vi "PLZ164WA_main.vi"() -> ()   [LabVIEW 2016]
doc: "Demonstrates the usage of major configuration controls. It configures the range, values, input and protection limits."
uses:
  <vilib>/Utility/file.llb/Read Delimited Spreadsheet (DBL).vi
  <instrlib>/Kikusui PLZ 4W Series/Kikusui PLZ 4W Series.lvlib
panel:
  in  "Stop VI":bool
  in  "file path":path=path "C:/Repository/bdc_prototype/logger/new_current_profile.csv"
  in  "Serial Configuration":cluster{"Baud Rate":u32, "Stop Bits":u16}={"Baud Rate"=19200, "Stop Bits"=20} {"Stop Bits" items=["1.0"=10, "2.0"=20]; "Baud Rate" items=["2400"=2400, "4800"=4800, "9600"=9600, "19200"=19200]}
  in  "OPP Trip (Disable)":bool=TRUE
  in  "OCP Trip (Disable)":bool=TRUE
  in  "UVP (Enable)":bool
  in  "Enable Input Short (Disable)":bool
  in  "Enable Input (Enable)":bool=TRUE
  in  "UVP Limit (0)":dbl
  in  "OPP Limit (0)":dbl=5.0
  in  "OCP Limit (0)":dbl=3.0
  in  "VISA resource name":refnum<visa-resource-name>="USB0::0x0B3E::0x1019::YL002399::INSTR"
  # "(c) 2009  National Instruments.  ALL RIGHTS RESERVED."
  # "Input Controls"
  # "Input Protection Controls"
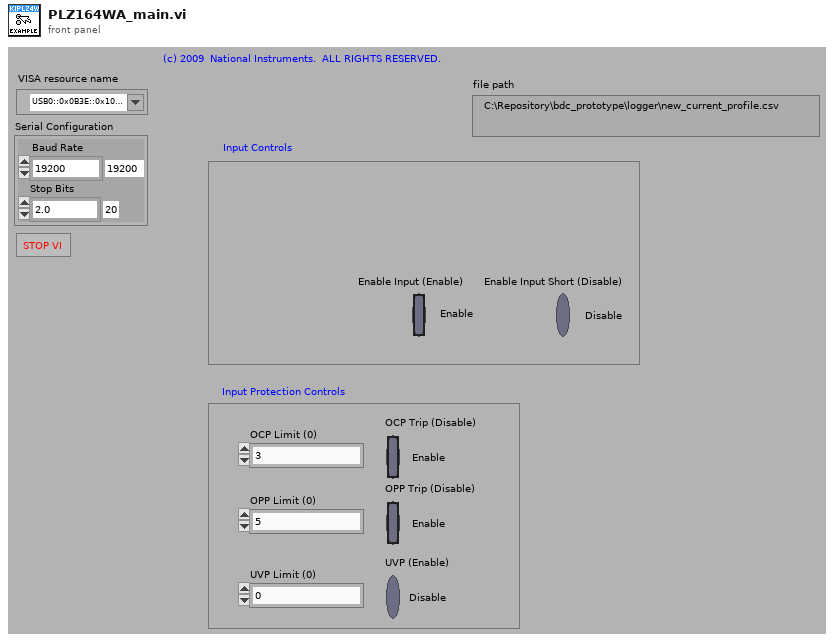
[diagram p1: front panel]
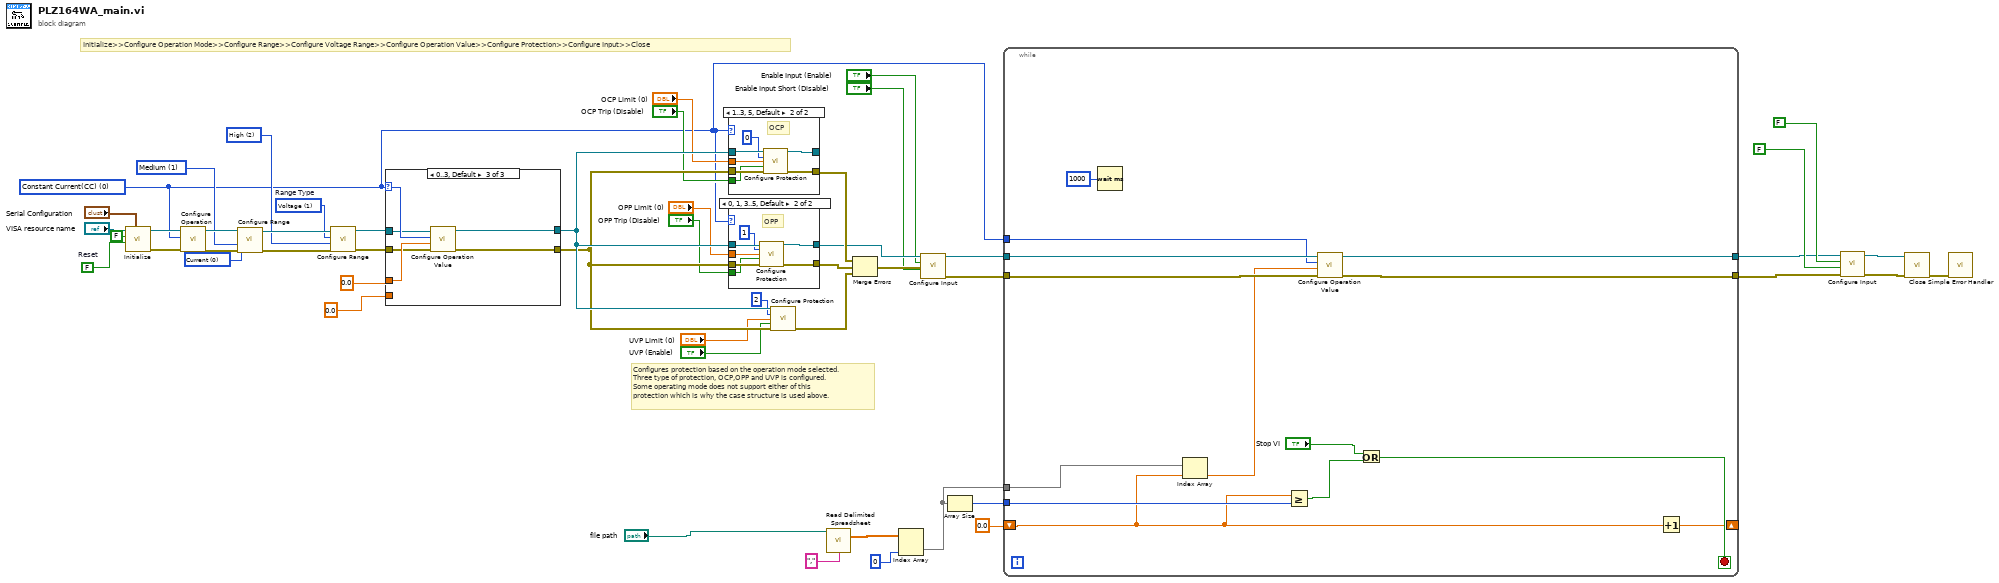
[diagram p0: block diagram]
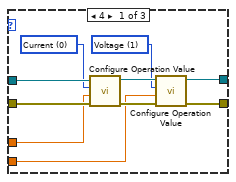
[diagram p4: hidden frame]
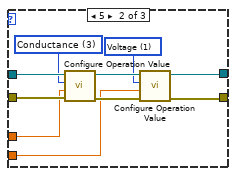
[diagram p5: hidden frame]
diagram:
  w2 = u16 0 items=["Current", "Voltage", "Power", "Conductance"] ("Range Type (0:Current)")
  w39 = u16 2 items=["Low"=0, "High"=2] ("Voltage Range (0:Low)")
  w38 = u16 1 items=["Low", "Medium", "High"] ("Input Range (0:Low)")
  w3 = u16 0 items=["Constant Current(CC)", "Constant Voltage(CV)", "Constant Power(CP)", "Constant Resistance(CR)", "Constant Current & Voltage(CCCV)", "Constant Resistance & Voltage(CRCV)"] ("Operation Mode (0:Constant Current)")
  w22 = FALSE  # Reset
  w40 = u16 1 items=["Current", "Voltage", "Power", "Conductance"]  # Range Type
  # "Configures protection based on the operation mode selected. Three type of protection, OCP,OPP and UVP is configured. Some operating mode does not support either of this protection which is why the case structure is used above."
  # "Initialize>>Configure Operation Mode>>Configure Range>>Configure Voltage Range>>Configure Operation Value>>Configure Protection>>Configure Input>>Close"
  n1 = call <instrlib>:"Initialize.vi"("Serial Configuration"="Serial Configuration", "Reset (True)"=w22, "ID Query (True)"=FALSE, "VISA resource name"="VISA resource name") -> ("error out"=w47:errorcluster, "VISA resource name out"=w48:refnum<visa-resource-name>)  [unwired: 6 in]
  n2 = call <instrlib>:"Configure Operation.vi"("error in (no error)"=w47, "Operation Mode (0:Constant Current)"=w3, "VISA resource name"=w48) -> ("error out"=w41:errorcluster, "VISA resource name out"=w42:refnum<visa-resource-name>)  [unwired: 7 in]
  n3 = call <instrlib>:"Configure Range.vi"("error in (no error)"=w41, "Range (0:Low)"=w38, "Range Type (0:Current)"=w2, "VISA resource name"=w42) -> ("error out"=w43:errorcluster, "VISA resource name out"=w44:refnum<visa-resource-name>)  [unwired: 6 in]
  n4 = call <instrlib>:"Configure Range.vi"("error in (no error)"=w43, "Range (0:Low)"=w39, "Range Type (0:Current)"=w40, "VISA resource name"=w44) -> ("error out"=w45:errorcluster, "VISA resource name out"=w46:refnum<visa-resource-name>)  [unwired: 6 in]
  n5 = case shown="0..3, Default" w3 {
    selector: w3 -> [_ _ w74]
    tunnel: 0.0 ("Input Value(0)") -> [w56 w64 w77]
    tunnel: w46 -> [w61 w69 w73]
    tunnel: w45 -> [w60 w68 w72]
    tunnel: [w57 w67 w76] -> w37
    tunnel: [w54 w66 w75] -> w36
    tunnel: 0.0 ("Voltage Value (0)") -> [w55 w65 _]
    frame 4 {
      w52 = u16 1 items=["Current", "Voltage", "Power", "Conductance"] ("Value Type (0:Current)")
      w53 = u16 0 items=["Current", "Voltage", "Power", "Conductance"] ("Value Type (0:Current)")
      n6 = call <instrlib>:"Configure Operation Value.vi"("error in (no error)"=w60, "Values (0)"=w56, "Value Type (0:Current)"=w53, "VISA resource name"=w61) -> ("error out"=w58:errorcluster, "VISA resource name out"=w59:refnum<visa-resource-name>)  [unwired: 6 in]
      n7 = call <instrlib>:"Configure Operation Value.vi"("error in (no error)"=w58, "Values (0)"=w55, "Value Type (0:Current)"=w52, "VISA resource name"=w59) -> ("error out"=w54:errorcluster, "VISA resource name out"=w57:refnum<visa-resource-name>)  [unwired: 6 in]
    }
    frame 5 {
      w62 = u16 1 items=["Current", "Voltage", "Power", "Conductance"] ("Value Type (0:Current)")
      w63 = u16 3 items=["Current", "Voltage", "Power", "Conductance"] ("Value Type (0:Current)")
      n8 = call <instrlib>:"Configure Operation Value.vi"("error in (no error)"=w68, "Values (0)"=w64, "Value Type (0:Current)"=w63, "VISA resource name"=w69) -> ("error out"=w70:errorcluster, "VISA resource name out"=w71:refnum<visa-resource-name>)  [unwired: 6 in]
      n9 = call <instrlib>:"Configure Operation Value.vi"("error in (no error)"=w70, "Values (0)"=w65, "Value Type (0:Current)"=w62, "VISA resource name"=w71) -> ("error out"=w66:errorcluster, "VISA resource name out"=w67:refnum<visa-resource-name>)  [unwired: 6 in]
    }
    frame 0..3, Default {
      n10 = call <instrlib>:"Configure Operation Value.vi"("error in (no error)"=w72, "Values (0)"=w77, "Value Type (0:Current)"=w74, "VISA resource name"=w73) -> ("error out"=w75:errorcluster, "VISA resource name out"=w76:refnum<visa-resource-name>)  [unwired: 6 in]
    }
  }
  n11 = case shown="1..3, 5, Default" w3 {
    tunnel: w37 -> [w79 w86]
    tunnel: w36 -> [w78 w85]
    tunnel: [w79 w84] -> _
    tunnel: [w78 w83] -> w35
    tunnel: "OCP Limit (0)" -> [_ w82]
    tunnel: "OCP Trip (Disable)" -> [_ w80]
    frame 0, 4 {
    }
    frame 1..3, 5, Default {
      # "OCP"
      n12 = call <instrlib>:"Configure Protection.vi"("VISA resource name"=w86, "Protection Type (0:OCP)"=0, "Protection Limit (0)"=w82, "Enable Trip (Disable)"=w80, "error in (no error)"=w85) -> ("VISA resource name out"=w84:refnum<visa-resource-name>, "error out"=w83:errorcluster)  [unwired: 9 in]
    }
  }
  n13 = case shown="0, 1, 3..5, Default" w3 {
    tunnel: w37 -> [w88 w95]
    tunnel: w36 -> [w87 w94]
    tunnel: [w88 w93] -> w32
    tunnel: [w87 w92] -> w24
    tunnel: "OPP Limit (0)" -> [_ w91]
    tunnel: "OPP Trip (Disable)" -> [_ w89]
    frame 2 {
    }
    frame 0, 1, 3..5, Default {
      # "OPP"
      n14 = call <instrlib>:"Configure Protection.vi"("VISA resource name"=w95, "Protection Type (0:OCP)"=1, "Protection Limit (0)"=w91, "Enable Trip (Disable)"=w89, "error in (no error)"=w94) -> ("VISA resource name out"=w93:refnum<visa-resource-name>, "error out"=w92:errorcluster)  [unwired: 9 in]
    }
  }
  n15 = call <instrlib>:"Configure Protection.vi"("VISA resource name"=w37, "Protection Type (0:OCP)"=2, "Protection Limit (0)"="UVP Limit (0)", "Enable Trip (Disable)"="UVP (Enable)", "error in (no error)"=w36) -> ("error out"=w34:errorcluster)  [unwired: 9 in, 1 out]
  n16 = call-poly <vilib>:"Read Delimited Spreadsheet.vi"("file path (dialog if empty)"="file path", "delimiter (\\t)"="," ("delimiter (\\t)")) -> ("all rows"=w7:dbl[][])  [unwired: 8 in, 5 out]
  n17 = Merge Errors(w35, w24, w34) -> (w33:errorcluster)
  n18 = Index Array(array=w7, index (col)=0 ("disabled index (col)")) -> (element=w5:dbl[])  [unwired: 1 in]
  n19 = call <instrlib>:"Configure Input.vi"("error in (no error)"=w33, "Enable Input Short (Disable)"="Enable Input Short (Disable)", "Enable Input (Enable)"="Enable Input (Enable)", "VISA resource name"=w32) -> ("error out"=w13:errorcluster, "VISA resource name out"=w14:refnum<visa-resource-name>)  [unwired: 6 in]
  n20 = Array Size(array=w5) -> (size(s)=w6:i32)
  n21 = while {
    tunnel: [w100] -> w12
    tunnel: w14 -> [w103]
    tunnel: [w101] -> w11
    tunnel: w13 -> [w102]
    tunnel: w6 -> [w107]
    tunnel: w5 -> [w104]
    shift-right: [w105] -> _
    shift-left: 0.0 -> [w97]
    tunnel: w3 -> [w99]
    stop <- w106 stop-if-true
    n22 = Wait (ms)(milliseconds to wait=u32 1000) -> ()  [unwired: 1 out]
    n23 = Index Array(array=w104, index=w97) -> (element=w98:dbl)
    n24 = Greater Or Equal?(x=w97, y=w107) -> (x >= y?=w109:bool)
    n25 = call <instrlib>:"Configure Operation Value.vi"("error in (no error)"=w102, "Values (0)"=w98, "Value Type (0:Current)"=w99, "VISA resource name"=w103) -> ("error out"=w101:errorcluster, "VISA resource name out"=w100:refnum<visa-resource-name>)  [unwired: 6 in]
    n26 = Or(x="Stop VI", y=w109) -> (x .or. y?=w106:bool)
    n27 = Increment(x=w97) -> (x+1=w105:dbl)
  }
  n28 = call <instrlib>:"Configure Input.vi"("error in (no error)"=w11, "Enable Input Short (Disable)"=FALSE ("Enable Input Short (Disable) 2"), "Enable Input (Enable)"=FALSE ("Enable Input (Enable) 2"), "VISA resource name"=w12) -> ("error out"=w15:errorcluster, "VISA resource name out"=w16:refnum<visa-resource-name>)  [unwired: 6 in]
  n29 = call <instrlib>:"Close.vi"("error in (no error)"=w15, "VISA resource name"=w16) -> ("error out"=w27:errorcluster)  [unwired: 9 in]
  n30 = call <vilib>:"Simple Error Handler.vi"("error in (no error)"=w27) -> ()  [unwired: 4 in, 5 out]
